vi "Connection Get Node.vi"(8 "error in (no error)":errorcluster, 10 "Path in":string, 11 "Connection DVR in":refnum<data-value>) -> (0 "error out":errorcluster, 2 "Node out":refnum<data-value>, 3 "Connection DVR out":refnum<data-value>)   [LabVIEW 2015, in "MDSplus.lvlib"]
uses:
  <vilib>/MDSplus_LV2015/Library/MDSplus.lvlib
  <vilib>/MDSplus_LV2015/Classes/Connection_Class/Connection.lvclass
  <vilib>/MDSplus_LV2015/Classes/Data_Class/TreeNode_Class/TreeNode.lvclass
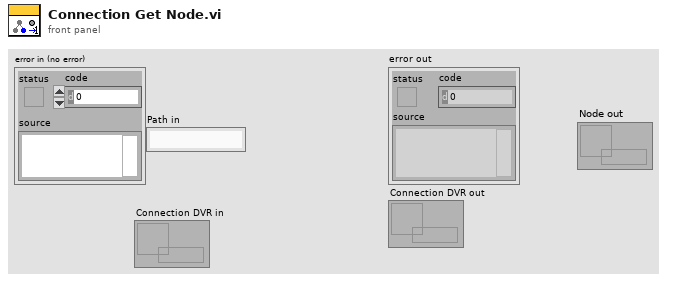
[diagram p1: front panel]
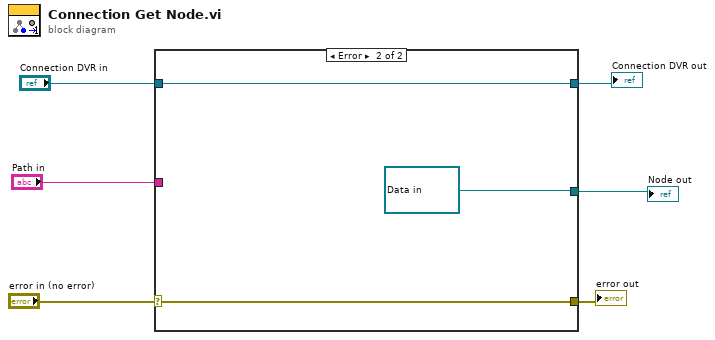
[diagram p0: block diagram]
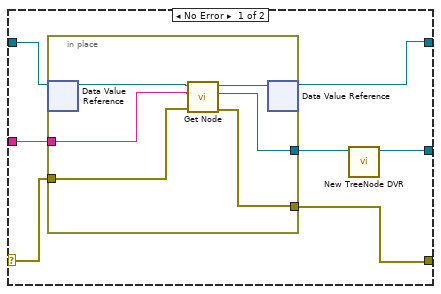
[diagram p2: hidden frame]
diagram:
  n1 = case shown="Error" "error in (no error)" {
    selector: "error in (no error)" -> [w10 w22]
    tunnel: [w8 w22] -> w5
    tunnel: "Connection DVR in" -> [w13 w21]
    tunnel: [w12 w21] -> w3
    tunnel: "Path in" -> [w11 _]
    tunnel: [w7 refnum<data-value> refnum ("TreeNode DVR out")] -> w1
    frame No Error {
      n2 = in-place {
        in-place-border: w11 -> [w17]
        in-place-border: w10 -> [w16]
        in-place-border: [w15] -> w8
        in-place-border: [w14] -> w9
        n3 = in-place-dvr #1(w13) -> (w19:refnum<class "Connection.lvclass">)  [unwired: 1 out]
        n4 = call <vilib>:"Get Node.vi"("error in (no error)"=w16, "Path in"=w17, "Connection in"=w19) -> ("error out"=w15:errorcluster, "Node out"=w14:refnum<class "TreeNode.lvclass">, "Connection out"=w18:refnum<class "Connection.lvclass">)  [unwired: 6 in]
        n5 = in-place-dvr #1(w18) -> (w12:refnum<data-value>)  [unwired: 1 out]
      }
      n6 = call <vilib>:"New TreeNode DVR.vi"("TreeNode in"=w9) -> ("TreeNode DVR out"=w7:refnum<data-value>)  [unwired: 9 in, 1 out]
    }
    frame Error {
    }
  }
  "error out" <- w5
  "Connection DVR out" <- w3
  "Node out" <- w1
